vi "CreateNewDataEvent.vi"(7 "Qbus":refnum<class "Qbus.lvclass">, 8 "error in (no error)":errorcluster, 9 "data flow":T7, 10 "data event config":T1, 11 "config":T10) -> (0 "error out":errorcluster, 3 "config out":T10)   [LabVIEW 2017, in "CmsDataEventCreator.lvlib"]
uses:
  <vilib>/addons/InsightCM/Devices/Shared/Cms/CmsDataEventCreator/CmsDataEventCreator.lvlib
  <vilib>/addons/InsightCM/Devices/Shared/Cms/CmsDataEventCreator/controls/config.ctl
  <vilib>/addons/Qbus/Qbus.lvclass
  <vilib>/addons/InsightCM/Devices/Shared/Common/DataFlow/controls/Data.ctl
  <vilib>/addons/InsightCM/Utilities/DataAccessors/controls/wfmSGL_DVR.ctl
  <vilib>/addons/PointValueMap/controls/PointMap.ctl
  <vilib>/addons/InsightCM/Devices/Shared/Common/DataFlow/controls/Type.ctl
  <vilib>/addons/InsightCM/Devices/Shared/Cms/CmsDataEventCreator/controls/DataEventConfig.ctl
  <vilib>/addons/InsightCM/Devices/Shared/Cms/CmsDataEventCreator/controls/AcqParams.ctl
  <vilib>/addons/InsightCM/Devices/Shared/Common/DataAccumulator/controls/AccumulationSettings.ctl
  <vilib>/addons/InsightCM/Devices/Shared/Common/DataAccumulator/controls/accumulationType.ctl
  <vilib>/addons/InsightCM/Devices/Shared/Common/DVRBuffer/controls/BufferLocation.ctl
  <vilib>/addons/InsightCM/Devices/Shared/Common/FileFlow/subVIs/GetFirstProcessModule_EventRef.vi
  <vilib>/addons/InsightCM/Devices/Shared/Common/FileFlow/FileFlow.lvlib
  <vilib>/addons/InsightCM/Devices/Shared/Common/DataEventCreator/DataEventCreator.lvlib
  <vilib>/addons/PointValueMap/PointValueMap.lvlib
  <vilib>/addons/InsightCM/Devices/Shared/Common/DataFlow/DataFlow.lvlib
  <vilib>/addons/InsightCM/Devices/Shared/Common/DataAccumulator/DataAccumulator.lvlib
  <vilib>/addons/InsightCM/Devices/Shared/Common/DVRBuffer/DVRBuffer.lvlib
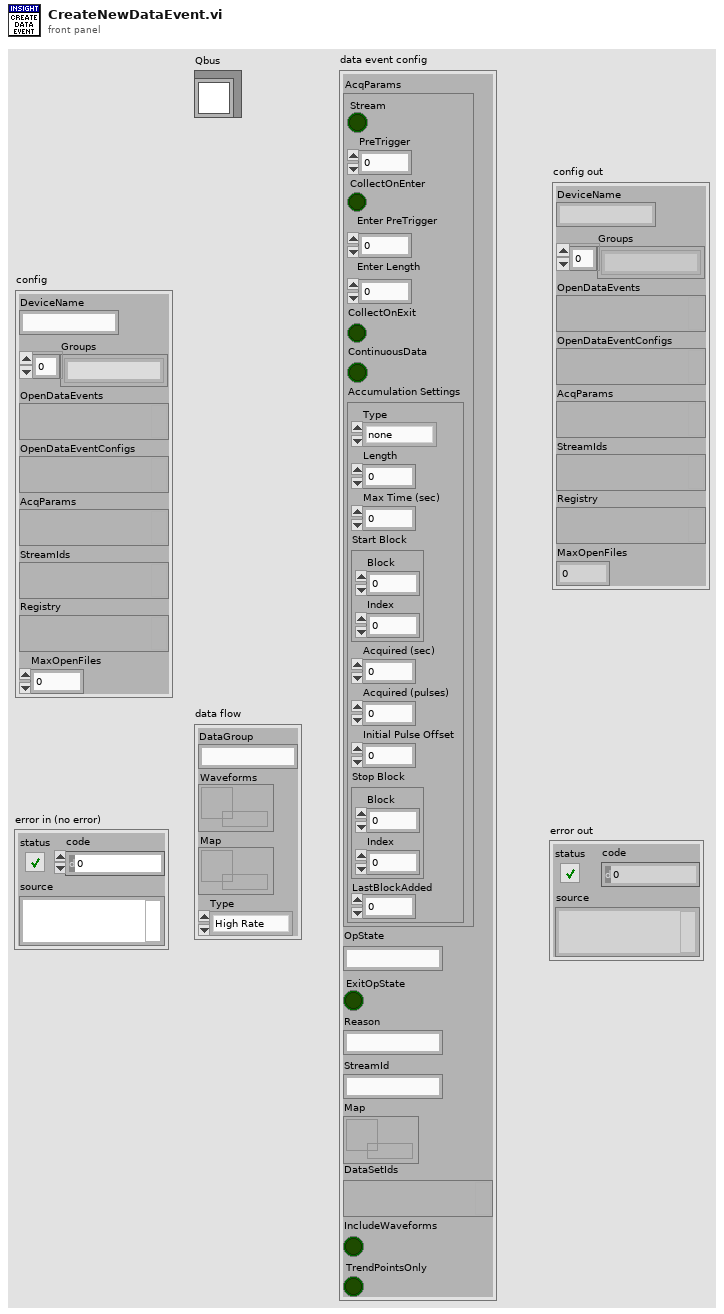
[diagram p1: front panel]
types:
  T1 = typedef "CmsDataEventCreator.lvlib/DataEventConfig.ctl" = cluster{"AcqParams":T2, "OpState":string, "ExitOpState":bool, "Reason":string, "StreamId":string, "Map":T6, "DataSetIds":variant, "IncludeWaveforms":bool, "TrendPointsOnly":bool}
  T2 = typedef "CmsDataEventCreator.lvlib/AcqParams.ctl" = cluster{"Stream":bool, "PreTrigger":i32, "CollectOnEnter":bool, "Enter PreTrigger":i32, "Enter Length":dbl, "CollectOnExit":bool, "ContinuousData":bool, "Accumulation Settings":T3}
  T3 = typedef "DataAccumulator.lvlib/AccumulationSettings.ctl" = cluster{"Type":T4, "Length":dbl, "Max Time (sec)":dbl, "Start Block":T5, "Acquired (sec)":dbl, "Acquired (pulses)":i32, "Initial Pulse Offset":dbl, "Stop Block":T5, "LastBlockAdded":u32}
  T4 = typedef "DataAccumulator.lvlib/accumulationType.ctl" = enum16{"none", "seconds", "revolutions"}
  T5 = typedef "DVRBuffer.lvlib/BufferLocation.ctl" = cluster{"Block":u32, "Index":i32}
  T6 = typedef "PointValueMap.lvlib/PointMap.ctl" = refnum<data-value>
  T7 = typedef "DataFlow.lvlib/Data.ctl" = cluster{"DataGroup":string, "Waveforms":T8, "Map":T6, "Type":T9}
  T8 = typedef "wfmSGL_DVR.ctl" = refnum<data-value>
  T9 = typedef "DataFlow.lvlib/Type.ctl" = enum16{"High Rate", "Low Rate", "Burst Mode"}
  T10 = typedef "CmsDataEventCreator.lvlib/config.ctl" = cluster{"DeviceName":string, "Groups":string[], "OpenDataEvents":variant, "OpenDataEventConfigs":variant, "AcqParams":variant, "StreamIds":variant, "Registry":variant, "MaxOpenFiles":i32}
  T11 = typedef "DataEvent.lvlib/Event.ctl" = cluster{"DataEvent":T12, "DataSets":T14[], "TrendPoints":T16[], "Alarms":T17[]}
  T12 = typedef "DataEvent.ctl" = cluster{"Id":string, "AssetNodeId":string, "Timestamp":i64, "Props":T13[]}
  T13 = typedef "KeyValuePair.ctl" = cluster{"Key":string, "Value":string}
  T14 = typedef "DataEvent.lvlib/DataSet.ctl" = cluster{"DataSetMetadata":T15, "Values":sgl[], "Values DVR":refnum<data-value>}
  T15 = typedef "DataSetMetadata.ctl" = cluster{"Id":string, "DataEventId":string, "AssetNodeId":string, "Type":string, "T0":i64, "Props":T13[]}
  T16 = typedef "TrendPoint.ctl" = cluster{"TrendPointId":string, "DataEventId":string, "Timestamp":i64, "Value":dbl, "Props":T13[]}
  T17 = typedef "TrendAlarmUpdate.ctl" = cluster{"RuleId":string, "Transition":T18}
  T18 = typedef "TrendAlarmTransition.ctl" = cluster{"At":i64, "Severity":i32, "Value":dbl, "Properties":T13[]}
  T19 = typedef "CmsDataEventCreator.lvlib/GroupRegistry.ctl" = cluster{"AssetNodeMap":variant, "DataSets":T20[], "Trends":T22[]}
  T20 = typedef "CmsDataEventCreator.lvlib/DataSetRegistry.ctl" = cluster{"ChannelName":string, "DataSetType":T21, "DoNotWriteToDB":bool, "ParentName":string, "CalculateOnServer":bool}
  T21 = typedef "DataEvent.lvlib/DataSetType.ctl" = enum16{"Waveform", "SpeedProfile", "ThermalImage", "EmsaSweep"}
  T22 = typedef "DataEventCreator.lvlib/Registry_Trend.ctl" = cluster{"TrendPointId":string, "DataSetName":string, "HighRate":bool, "Always Send":bool}
  T23 = typedef "FileFlow.lvlib/data_eventRef.ctl" = cluster{"event reference":T24, "DataGroup":string, "OperatingState":string, "StreamId":string, "LastBlock":bool, "Map":T6, "TrendPoints Only":bool, "Extra Large File":bool}
  T24 = typedef "DataEvent.lvlib/EventReference.ctl" = refnum<data-value>
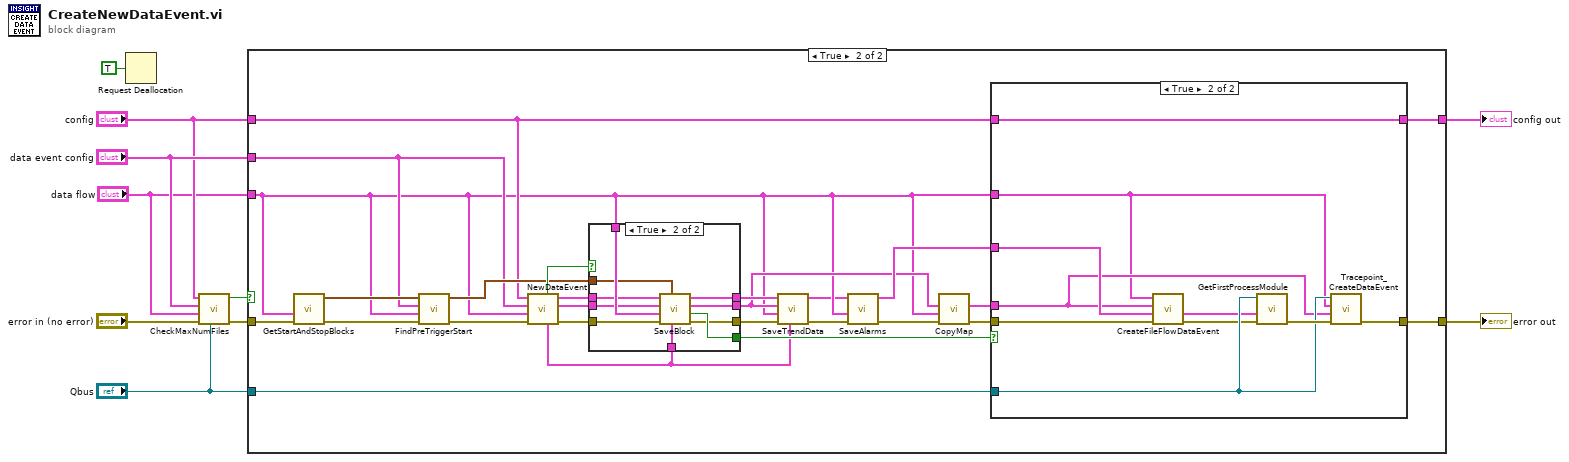
[diagram p0: block diagram]
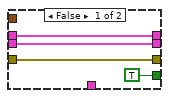
[diagram p3: hidden frame]
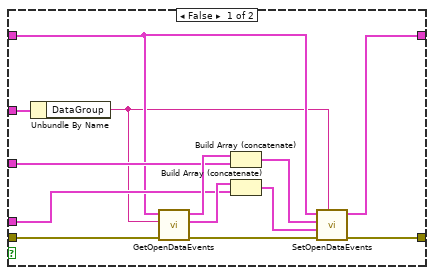
[diagram p4: hidden frame]
diagram:
  n1 = Request Deallocation(TRUE ("flag")) -> ()
  n2 = call <vilib>:"CheckMaxNumFiles.vi"("Qbus"="Qbus", "error in (no error)"="error in (no error)", "data"="data flow", "data event config"="data event config", "config"="config") -> ("error out"=w7:errorcluster, "ok to open new file"=w4:bool)  [unwired: 5 in]
  n3 = case shown="True" w4 {
    tunnel: "data flow" -> [_ w14]
    tunnel: w7 -> [w11 w38]
    tunnel: "config" -> [w12 w26]
    tunnel: [w12 w28] -> w10
    tunnel: "Qbus" -> [_ w34]
    tunnel: [w11 w36] -> w9
    tunnel: "data event config" -> [_ w19]
    frame False {
    }
    frame True {
      n4 = call <vilib>:"GetStartAndStopBlocks.vi"("error in (no error)"=w38, "data"=w14) -> ("error out"=w37:errorcluster, "start block"=w31:T5)  [unwired: 7 in, 1 out]
      n5 = call <vilib>:"FindPreTriggerStart.vi"("error in (no error)"=w37, "data"=w14, "data event"=w19, "start block"=w31) -> ("error out"=w20:errorcluster, "pretrigger start"=w27:T5)  [unwired: 4 in, 2 out]
      n6 = call <vilib>:"NewDataEvent.vi"("error in (no error)"=w20, "data flow"=w14, "data event"=w19, "config"=w26) -> ("error out"=w22:errorcluster, "data event config"=w25:T1, "data event"=w18:T11, "registry"=w21:T19, "save waveforms"=w30:bool)  [unwired: 3 in]
      n7 = case shown="True" w30 {
        tunnel: w22 -> [w41 w47]
        tunnel: [w41 w46] -> w33
        tunnel: [TRUE ("file complete") w49] -> w32
        tunnel: w25 -> [w40 w45]
        tunnel: w14 -> [_ w52]
        tunnel: w21 -> [_ w51]
        tunnel: w27 -> [_ w50]
        tunnel: [w40 w48] -> w15
        tunnel: [w39 w44] -> w16
        tunnel: w18 -> [w39 w43]
        frame False {
        }
        frame True {
          n8 = call <vilib>:"SaveBlock.vi"("Registry"=w51, "start block"=w50, "error in (no error)"=w47, "data"=w52, "data event config"=w45, "data event"=w43) -> ("error out"=w46:errorcluster, "file complete"=w49:bool, "data event config out"=w48:T1, "data event out"=w44:T11)  [unwired: 2 in]
        }
      }
      n9 = call <vilib>:"SaveTrendData.vi"("registry"=w21, "error in (no error)"=w33, "data"=w14, "data event config"=w15, "data event"=w16) -> ("error out"=w24:errorcluster, "data event out"=w13:T11)  [unwired: 5 in]
      n10 = call <vilib>:"SaveAlarms.vi"("error in (no error)"=w24, "data flow"=w14, "data event"=w13) -> ("error out"=w23:errorcluster, "data event out"=w17:T11)  [unwired: 7 in]
      n11 = call <vilib>:"CopyMap.vi"("error in (no error)"=w23, "data"=w14, "data event config"=w15) -> ("error out"=w35:errorcluster, "data event config out"=w29:T1)  [unwired: 7 in]
      n12 = case shown="True" w32 {
        tunnel: w35 -> [w53 w70]
        tunnel: w29 -> [w61 w67]
        tunnel: w34 -> [_ w72]
        tunnel: [w54 w73] -> w36
        tunnel: w26 -> [w60 w75]
        tunnel: [w55 w75] -> w28
        tunnel: w14 -> [w65 w66]
        tunnel: w17 -> [w62 w68]
        frame False {
          n13 = Unbundle By Name(w65) -> ("DataGroup"=w56:string)
          n14 = call <vilib>:"GetOpenDataEvents.vi"("error in (no error)"=w53, "data group"=w56, "config"=w60) -> ("error out"=w57:errorcluster, "open data event configs"=w63:T1[], "open data events"=w64:T11[])  [unwired: 6 in]
          n15 = Build Array (concatenate)(w64, w62) -> (w59:T11[])
          n16 = Build Array (concatenate)(w63, w61) -> (w58:T1[])
          n17 = call <vilib>:"SetOpenDataEvents.vi"("data group"=w56, "error in (no error)"=w57, "data event configs"=w58, "data events"=w59, "config"=w60) -> ("error out"=w54:errorcluster, "config out"=w55:T10)  [unwired: 5 in]
        }
        frame True {
          n18 = call <vilib>:"CreateFileFlowDataEvent.vi"("error in (no error)"=w70, "data event"=w68, "data event config"=w67, "data flow"=w66) -> ("error out"=w69:errorcluster, "data event ref"=w71:T23)  [unwired: 6 in]
          n19 = call-poly <vilib>:"GetFirstProcessModule.vi"("error in (no error)"=w69, "data"=w71, "Qbus in"=w72) -> ("error out"=w74:errorcluster)  [unwired: 7 in, 1 out]
          n20 = call <vilib>:"Tracepoint_CreateDataEvent.vi"("error in (no error)"=w74, "data event"=w67, "data"=w66, "Qbus"=w72) -> ("error out"=w73:errorcluster)  [unwired: 7 in]
        }
      }
    }
  }
  "error out" <- w9
  "config out" <- w10
